vi "Find Edge Boundaries.vi"(0 "Amplitude Array":dbl[](array[numeric]), 1 "Low Level":dbl, 2 "High Level":dbl, 7 "Midpoint Index":dbl, 9 "Threshold % (10%)":dbl=10.0 min=0.0 max=100.0, 11 "Error In":errorcluster, 12 "Edge Direction":enum16{"Falling Edge", "Rising Edge"}(ring)) -> (4 "Edge Start Index":dbl, 6 "Edge Start":dbl, 8 "Edge End Index":dbl, 10 "Edge End":dbl, 15 "Error Out":errorcluster)   [LabVIEW 2021, in "Fits.lvlib"]
uses:
  Fits.lvlib
  Math/Math.lvlib
  Arrays/Arrays.lvlib
panel:
  out "Edge Low":dbl
  out "Edge High":dbl
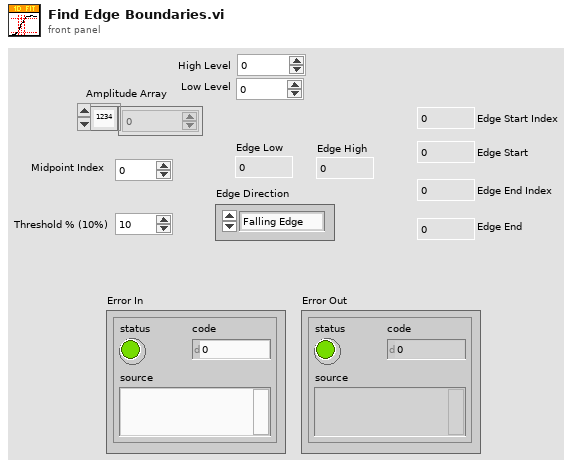
[diagram p1: front panel]
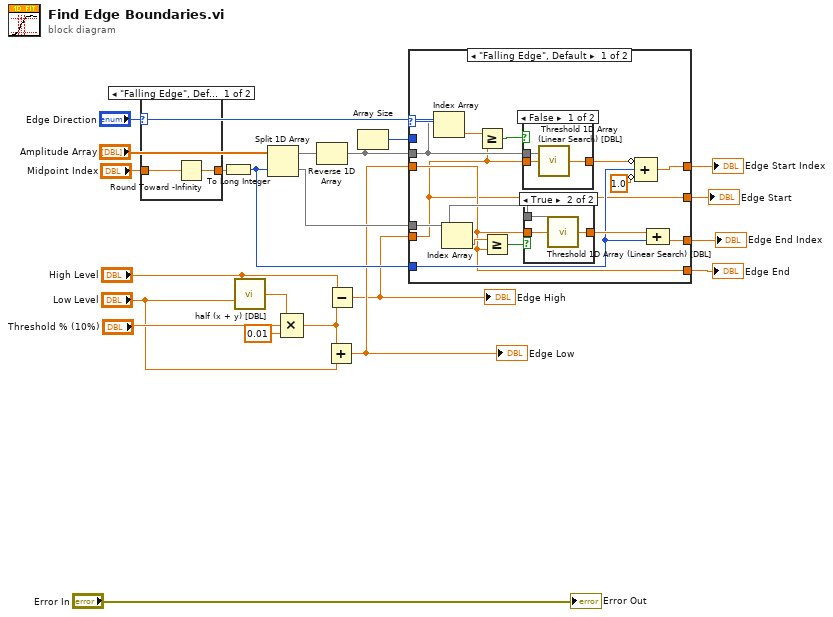
[diagram p0: block diagram]
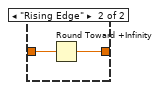
[diagram p2: hidden frame]
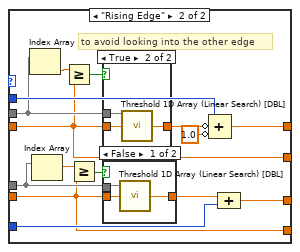
[diagram p5: hidden frame]
diagram:
  n1 = case shown="\"Falling Edge\", Default" "Edge Direction" {
    tunnel: "Midpoint Index" -> [w24 w26]
    tunnel: [w23 w25] -> w1
    frame "Falling Edge", Default {
      n2 = Round Toward -Infinity(1:w24) -> (0:w23:dbl)
    }
    frame "Rising Edge" {
      n3 = Round Toward +Infinity(x=w26) -> (ceil(x): smallest int >= x=w25:dbl)
    }
  }
  n4 = To Long Integer(number=w1) -> (32bit integer=w12:i32)
  n5 = call "half (x + y) [DBL].vi"("y"="Low Level", "x"="High Level") -> ("(x+y)/2"=w21:dbl)  [unwired: 4 in]
  n6 = Split 1D Array(array="Amplitude Array", index=w12) -> (first subarray=w15:dbl[], second subarray=w14:dbl[])
  n7 = Compound Arithmetic op=MULTIPLY(w21, "Threshold % (10%)", 0.01 ("value")) -> (w17:dbl)
  n8 = Reverse 1D Array(array=w15) -> (reversed array=w5:dbl[])
  n9 = Add(x=w17, y="Low Level") -> (x+y=w11:dbl)
  "Edge Low" <- w11
  n10 = Subtract(x="High Level", y=w17) -> (x-y=w10:dbl)
  "Edge High" <- w10
  n11 = Array Size(array=w5) -> (size(s)=w4:i32)
  n12 = case shown="\"Falling Edge\", Default" "Edge Direction" {
    tunnel: w5 -> [w30 w54]
    tunnel: w14 -> [w34 w50]
    tunnel: w12 -> [w36 w60]
    tunnel: w11 -> [w32 w52]
    tunnel: w10 -> [w28 w48]
    tunnel: [w37 w57] -> w9
    tunnel: [w38 w58] -> w8
    tunnel: [w28 w52] -> w7
    tunnel: [w32 w48] -> w6
    tunnel: w4 -> [_ w56]
    frame "Falling Edge", Default {
      n13 = Index Array(array=w30) -> (element=w29:dbl)  [unwired: 1 in]
      n14 = Index Array(array=w34) -> (element=w33:dbl)  [unwired: 1 in]
      n15 = Greater Or Equal?(x=w29, y=w28) -> (x >= y?=w27:bool)
      n16 = Greater Or Equal?(x=w33, y=w32) -> (x >= y?=w31:bool)
      n17 = case shown="False" w27 {
        tunnel: [w43 _] -> w40
        tunnel: w28 -> [w42 _]
        tunnel: w30 -> [w41 _]
        frame False {
          n18 = call "Threshold 1D Array (Linear Search) [DBL].vi"("Array"=w41, "Y"=w42) -> ("fractional index"=w43:dbl)  [unwired: 7 in]
        }
        frame True {
        }
      }
      n19 = case shown="True" w31 {
        tunnel: [_ w46] -> w39
        tunnel: w34 -> [_ w45]
        tunnel: w32 -> [_ w44]
        frame False {
        }
        frame True {
          n20 = call "Threshold 1D Array (Linear Search) [DBL].vi"("Array"=w45, "Y"=w44) -> ("fractional index"=w46:dbl)  [unwired: 7 in]
        }
      }
      n21 = Compound Arithmetic op=ADD(invert w40, w36, invert 1.0 ("value")) -> (w37:dbl)
      n22 = Compound Arithmetic op=ADD(w39, w36) -> (w38:dbl)
    }
    frame "Rising Edge" {
      # "to avoid looking into the other edge"
      n23 = Index Array(array=w54) -> (element=w53:dbl)  [unwired: 1 in]
      n24 = Index Array(array=w50) -> (element=w49:dbl)  [unwired: 1 in]
      n25 = Greater Or Equal?(x=w53, y=w52) -> (x >= y?=w51:bool)
      n26 = Greater Or Equal?(x=w49, y=w48) -> (x >= y?=w47:bool)
      n27 = case shown="True" w51 {
        tunnel: [_ w67] -> w59
        tunnel: w54 -> [_ w66]
        tunnel: w52 -> [_ w65]
        frame False {
        }
        frame True {
          n28 = call "Threshold 1D Array (Linear Search) [DBL].vi"("Array"=w66, "Y"=w65) -> ("fractional index"=w67:dbl)  [unwired: 7 in]
        }
      }
      n29 = case shown="False" w47 {
        tunnel: w50 -> [w64 _]
        tunnel: [w63 _] -> w61
        tunnel: w48 -> [w62 _]
        frame False {
          n30 = call "Threshold 1D Array (Linear Search) [DBL].vi"("Array"=w64, "Y"=w62) -> ("fractional index"=w63:dbl)  [unwired: 7 in]
        }
        frame True {
        }
      }
      n31 = Compound Arithmetic op=ADD(w56, invert w59, invert 1.0 ("value")) -> (w57:dbl)
      n32 = Compound Arithmetic op=ADD(w61, w60) -> (w58:dbl)
    }
  }
  "Edge End Index" <- w8
  "Edge Start Index" <- w9
  "Edge Start" <- w7
  "Edge End" <- w6
  "Error Out" <- "Error In"
